vi "Lift PID Control for tester.vi"(0 "Motors DevRefs IN":T10, 1 "Limit Switches":T14, 5 "Operator Gamepad":T18, 7 "Lift Potentionmeter":T15, 9 "Lift Deadband":dbl=0.1, 11 "Gains UP":cluster{"P":dbl, "I":dbl, "D":dbl}={"P"=0.1, "I"=0.0, "D"=0.0}, 12 "Gains DOWN":cluster{"P":dbl, "I":dbl, "D":dbl}={"P"=0.1, "I"=0.0, "D"=0.0}, 13 "Limit":dbl=0.666, 14 "Time to Wait":i32=10) -> (4 "Motor DevRefs OUT":T20, 10 "Tolerable?":bool)   [LabVIEW 2014]
uses:
  <vilib>/Rock Robotics/WPI/MotorControl/WPI_MotorControlDeviceRef.ctl
  <vilib>/Rock Robotics/WPI/MotorControl/WPI_MotorControlType.ctl
  <vilib>/Rock Robotics/SystemInterfaces/Typedef/FPGA_TypedefDigitalModule.ctl
  <vilib>/Rock Robotics/SystemInterfaces/DIO/FPGA_DIOPWMChannel.ctl
  <vilib>/Rock Robotics/WPI/PWM/WPI_PWMDeadband.ctl
  <vilib>/Rock Robotics/WPI/CAN/Jaguar/SubVIs/WPI_CANJaguar_ControlMode.ctl
  <vilib>/Rock Robotics/WPI/CAN/TalonSRX/WPI_CANTalonSRX_APIControlMode.ctl
  <vilib>/Rock Robotics/WPI/PWM/WPI_PWMTransform_ConPane.ctl
  <vilib>/Rock Robotics/WPI/Joystick/WPI_JoystickDevRef.ctl
  <vilib>/Rock Robotics/WPI/Joystick/WPI_JoystickDeviceEnum.ctl
  <vilib>/Rock Robotics/WPI/Potentiometer/WPI_PotentiometerDevRef.ctl
  <vilib>/Rock Robotics/SystemInterfaces/Typedef/FPGA_TypedefAnalogModule.ctl
  <vilib>/Rock Robotics/SystemInterfaces/AI/FPGA_AIChannel.ctl
  <vilib>/Rock Robotics/WPI/Switch/WPI_SwitchDevRef.ctl
  <vilib>/Rock Robotics/SystemInterfaces/DIO/FPGA_DIOChannel.ctl
  <vilib>/Rock Robotics/SystemInterfaces/Counter/FPGA_CounterCtrSystemIndex.ctl
  <vilib>/Rock Robotics/WPI/DriverStation/WPI_DriverStationRobotMode2.ctl
  Robot Global Data.vi
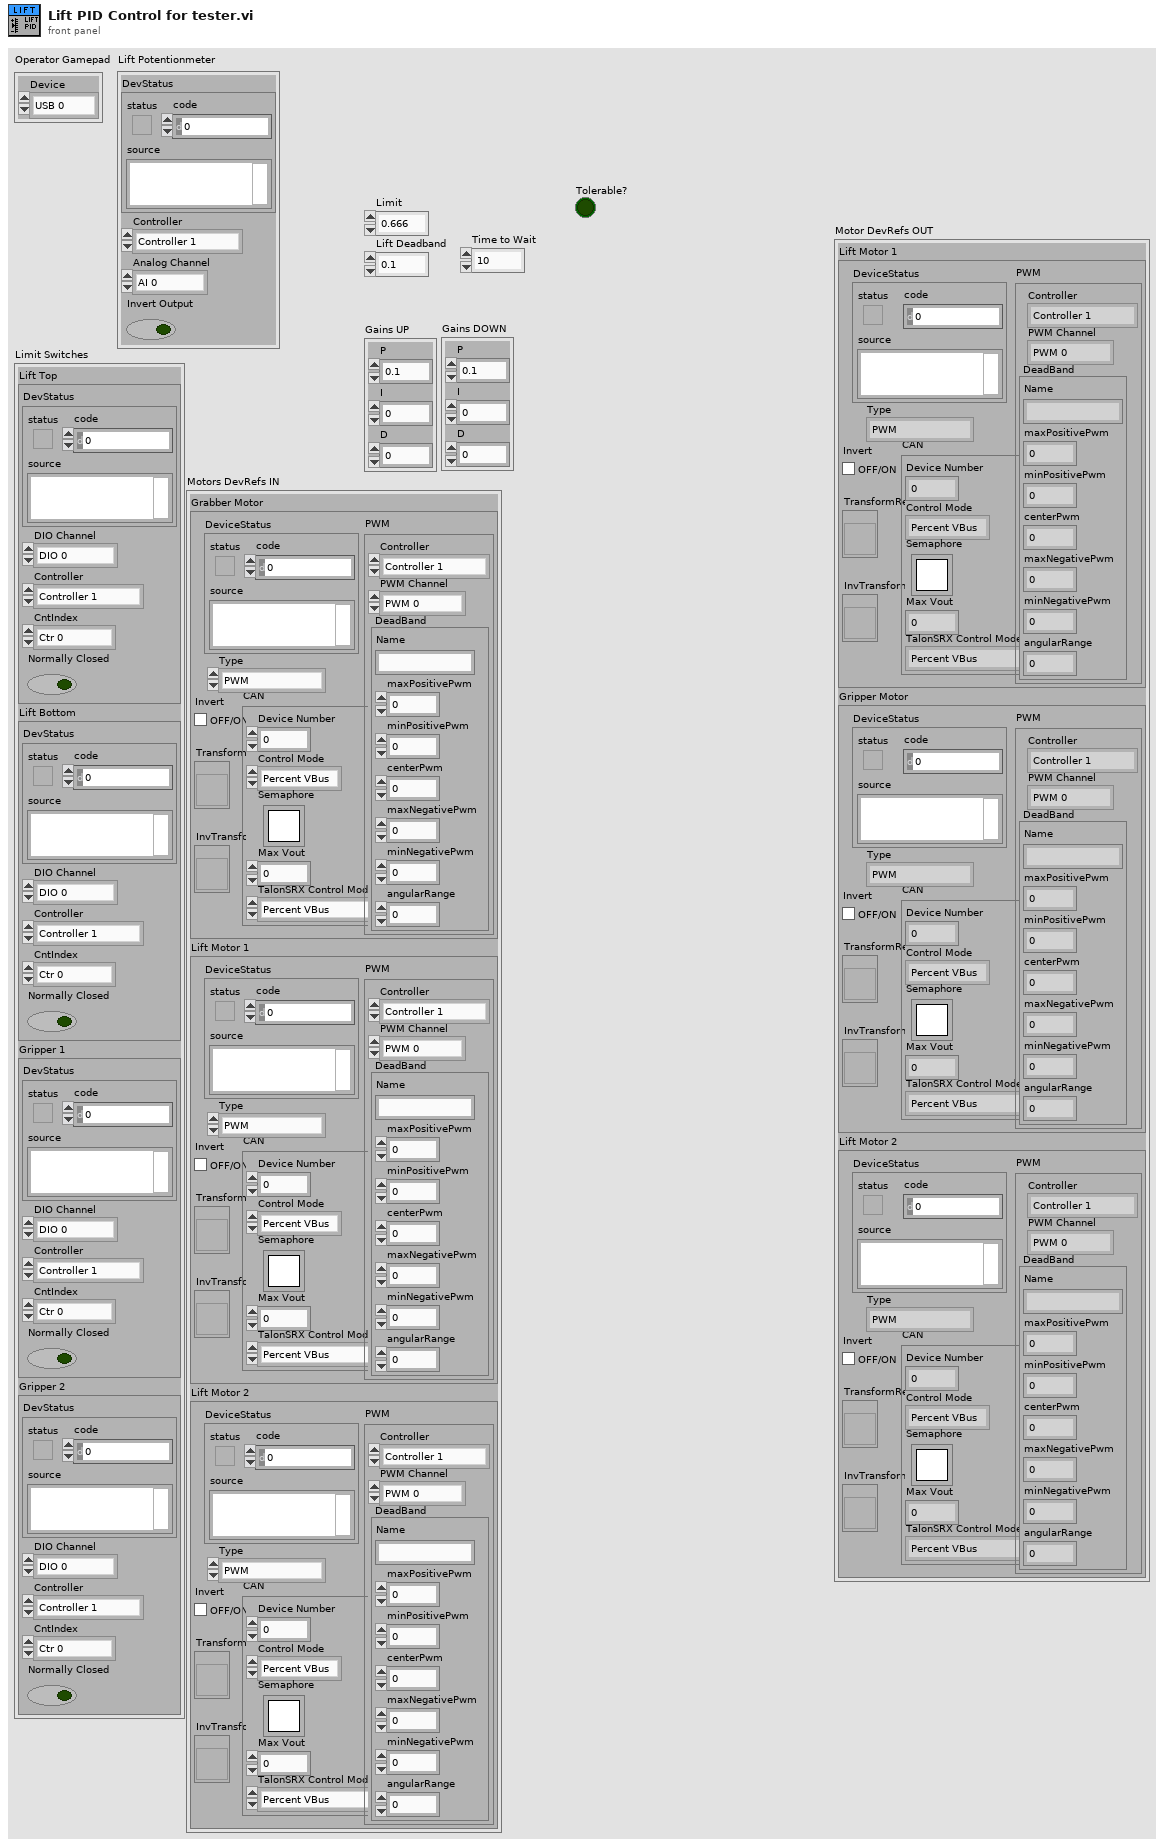
[diagram p1: front panel]
types:
  T1 = typedef "WPI_MotorControlDeviceRef.ctl" = cluster{"DeviceStatus":errorcluster, "Type":T2, "PWM":cluster{"Controller":T3, "PWM Channel":T4, "DeadBand":T5}, "CAN":cluster{"Device Number":u8, "Control Mode":T6, "Semaphore":T7, "Max Vout":dbl, "TalonSRX Control Mode":T8}, "Invert":bool, "TransformRef":T9, "InvTransformRef":T9}
  T2 = typedef "WPI_MotorControlType.ctl" = enum16{"PWM", "CAN", "CANTalonSRX"}
  T3 = typedef "FPGA_TypedefDigitalModule.ctl" = enum16{"Controller 1"}
  T4 = typedef "FPGA_DIOPWMChannel.ctl" = enum8{"PWM 0", "PWM 1", "PWM 2", "PWM 3", "PWM 4", "PWM 5", "PWM 6", "PWM 7", "PWM 8", "PWM 9", "PWM MXP 0", "PWM MXP 1", "PWM MXP 2", "PWM MXP 3", "PWM MXP 4", "PWM MXP 5", "PWM MXP 6", "PWM MXP 7", "PWM MXP 8", "PWM MXP 9", "Invalid"}
  T5 = typedef "WPI_PWMDeadband.ctl" = cluster{"Name":string, "maxPositivePwm":i32, "minPositivePwm":i32, "centerPwm":i32, "maxNegativePwm":i32, "minNegativePwm":i32, "angularRange":u16}
  T6 = typedef "WPI_CANJaguar_ControlMode.ctl" = enum8{"Percent VBus", "Current", "Speed", "Position", "Voltage"}
  T7 = typedef "Semaphore RefNum" = refnum<k1>
  T8 = typedef "WPI_CANTalonSRX_APIControlMode.ctl" = enum8{"Percent VBus", "Speed", "Position", "Slave", "Unchanged / Invalid"}
  T9 = typedef "WPI_PWMTransform_ConPane.ctl" = refnum<vi>
  T10 = cluster{"Grabber Motor":T1, "Lift Motor 1":T1, "Lift Motor 2":T1}
  T11 = typedef "WPI_SwitchDevRef.ctl" = cluster{"DevStatus":errorcluster, "DIO Channel":T12, "Controller":T3, "CntIndex":T13, "Normally Closed":bool}
  T12 = typedef "FPGA_DIOChannel.ctl" = enum8{"DIO 0", "DIO 1", "DIO 2", "DIO 3", "DIO 4", "DIO 5", "DIO 6", "DIO 7", "DIO 8", "DIO 9", "DIO MXP 0", "DIO MXP 1", "DIO MXP 2", "DIO MXP 3", "DIO MXP 4", "DIO MXP 5", "DIO MXP 6", "DIO MXP 7", "DIO MXP 8", "DIO MXP 9", "DIO MXP 10", "DIO MXP 11", "DIO MXP 12", "DIO MXP 13", "DIO MXP 14", "DIO MXP 15", "Invalid"}
  T13 = typedef "FPGA_CounterCtrSystemIndex.ctl" = enum8{"Ctr 0", "Ctr 1", "Ctr 2", "Ctr 3", "Ctr 4", "Ctr 5", "Ctr 6", "Ctr 7", "Invalid"}
  T14 = cluster{"Lift Top":T11, "Lift Bottom":T11, "Gripper 1":T11, "Gripper 2":T11}
  T15 = typedef "WPI_PotentiometerDevRef.ctl" = cluster{"DevStatus":errorcluster, "Controller":T16, "Analog Channel":T17, "Invert Output":bool}
  T16 = typedef "FPGA_TypedefAnalogModule.ctl" = enum16{"Controller 1"}
  T17 = typedef "FPGA_AIChannel.ctl" = enum8{"AI 0", "AI 1", "AI 2", "AI 3", "AI MXP 0", "AI MXP 1", "AI MXP 2", "AI MXP 3", "Invalid"}
  T18 = typedef "WPI_JoystickDevRef.ctl" = cluster{"Device":T19}
  T19 = typedef "WPI_JoystickDeviceEnum.ctl" = enum16{"USB 0", "USB 1", "USB 2", "USB 3", "USB 4", "USB 5"}
  T20 = cluster{"Lift Motor 1":T1, "Gripper Motor":T1, "Lift Motor 2":T1}
  T21 = typedef "WPI_DriverStationRobotMode2.ctl" = enum16{"Autonomous Disabled", "Autonomous Enabled", "Teleop Disabled", "Teleop Enabled", "Disconnected", "Finish", "Test Disabled", "Test Enabled", "Emergency Stopped"}
  T22 = cluster{"Error":dbl, "millisecond timer value":u32, "To Shift Register":dbl}
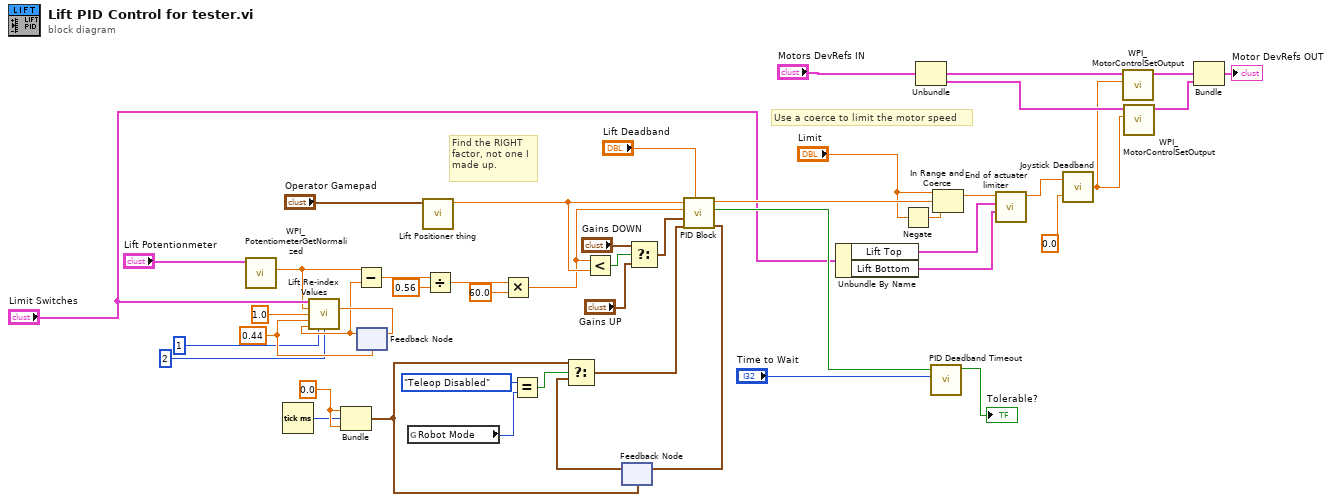
[diagram p0: block diagram]
diagram:
  w6 = 0.44 ("y")
  w32 = 0.0
  # "Find the RIGHT\nfactor, not one I\nmade up."
  # "Use a coerce to limit the motor speed"
  n1 = call <vilib>:"WPI_PotentiometerGetNormalized.vi"("PotDevRef"="Lift Potentionmeter") -> ("Normalized Value"=w8:dbl)  [unwired: 8 in, 2 out]
  n2 = Tick Count (ms)() -> (millisecond timer value=w31:u32)
  n3 = Bundle(w32, "millisecond timer value"=w31, w32) -> (w28:cluster{dbl, "millisecond timer value":u32, dbl})  [unwired: 1 in]
  n4 = feedback #1(w6) -> (w9:dbl)
  n5 = call "Lift Re-index Values.vi"("Limit Switches"="Limit Switches", "Input for Re-indexing"=w8, "Initial Upper Value"=1.0, "Initial Lower Value"=w6, "Current Lower Value"=w9, "Upper Limit Index ( 0 - 3 )"=1 ("Upper Limit Index ( 1 - 4 )"), "Lower Limit Index ( 0 - 3 )"=2 ("Upper Limit Index ( 1 - 4 )")) -> ("Re-indexed Value"=w10:dbl)  [unwired: 8 in]
  n6 = Subtract(x=w8, y=w9) -> (x-y=w19:dbl)
  n7 = feedback-in #1(w10) -> ()
  n8 = global read "Robot Global Data.vi" "Robot Mode"() -> (w25:T21)
  n9 = call "Lift Positioner thing.vi"("Operator Gamepad"="Operator Gamepad") -> ("Setpoint"=w12:dbl)  [unwired: 10 in]
  n10 = Divide(x=w19, y=0.56) -> (x/y=w3:dbl)
  n11 = Multiply(x=w3, y=60.0) -> (x*y=w2:dbl)
  n12 = Equal?(x=WPI_DriverStationRobotMode2."Teleop Disabled", y=w25) -> (x = y?=w27:bool)
  n13 = Less?(x=w2, y=w12) -> (x < y?=w13:bool)
  n14 = feedback #2(w28) -> (w29:cluster{dbl, "millisecond timer value":u32, dbl})
  n15 = Select(t=w28, s=w27, f=w29) -> (s? t:f=w30:cluster{dbl, "millisecond timer value":u32, dbl})
  n16 = Select(t="Gains DOWN", s=w13, f="Gains UP") -> (s? t:f=w16:cluster{"P":dbl, "I":dbl, "D":dbl})
  n17 = call "PID Block.vi"("Deadband"="Lift Deadband", "From Shift"=w30, "Gains"=w16, "Position"=w2, "Setpoint"=w12) -> ("To Shift"=w46:T22, "Tolerable?"=w45:bool, "Output"=w39:dbl)  [unwired: 4 in]
  n18 = feedback-in #2(w46) -> ()
  n19 = Unbundle By Name("Limit Switches") -> ("Lift Top"=w33:T11, "Lift Bottom"=w34:T11)
  n20 = Negate(x="Limit") -> (-x=w37:dbl)
  n21 = Unbundle("Motors DevRefs IN") -> ("Lift Motor 1"=w24:T1, "Lift Motor 2"=w43:T1)  [unwired: 1 out]
  n22 = call "PID Deadband Timeout.vi"("Time to Wait"="Time to Wait", "In deadband range?"=w45) -> ("Deadband Timed-out"=→"Tolerable?":bool)  [unwired: 9 in]
  n23 = In Range and Coerce(upper limit="Limit", x=w39, lower limit=w37) -> (coerced(x)=w38:dbl)  [unwired: 1 out]
  n24 = call "End of actuater limiter.vi"("Lower limit switch"=w34, "Upper limit switch"=w33, "Motor input"=w38) -> ("Motor output"=w18:dbl)  [unwired: 8 in]
  n25 = call "Joystick Deadband.vi"("Deadband"=0.0, "Joystick Value"=w18) -> ("Joystick Output"=w21:dbl)
  n26 = call <vilib>:"WPI_MotorControlSetOutput.vi"("Output"=w21, "MotorControlDevRef"=w24) -> ("MotorControlDevRef"=w22:T1)  [unwired: 7 in, 2 out]
  n27 = call <vilib>:"WPI_MotorControlSetOutput.vi"("Output"=w21, "MotorControlDevRef"=w43) -> ("MotorControlDevRef"=w42:T1)  [unwired: 7 in, 2 out]
  n28 = Bundle(cluster="Motors DevRefs IN", "Lift Motor 1"=w22, "Lift Motor 2"=w42) -> ()  [unwired: 1 in, 1 out]
  "Motor DevRefs OUT" <- "Motors DevRefs IN"
